vi "Format StateReasonType_LVXML.vi"(8 "error in (no error)":errorcluster, 10 "xmlData in":T2, 11 "AWS_EC2 in":refnum<class "AWS_EC2.lvclass">) -> (0 "error out":errorcluster, 2 "StateReasonType":T3, 3 "AWS_EC2 out":refnum<class "AWS_EC2.lvclass">)   [LabVIEW 2014, in "AWS_EC2.lvlib" / "AWS_EC2.lvclass"]
uses:
  AWS_EC2.lvclass
  EC2 Datatypes/StateReasonType.ctl
  lv-xml-parser/r0/trunk/VI Source/EventType.ctl
  AWS_EC2.lvlib
  lv-xml-parser/r0/trunk/VI Source/LV XML Parser.lvlib
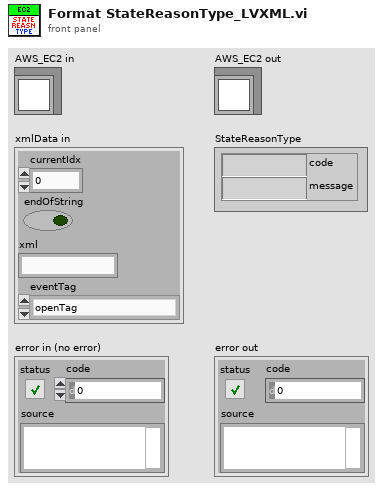
[diagram p1: front panel]
types:
  T1 = typedef "LV XML Parser.lvlib/EventType.ctl" = enum16{"openTag", "endOpenTag", "closeTag", "comment", "endComment", "endOfFile", "attribute", "startXml"}
  T2 = cluster{"currentIdx":i32, "endOfString":bool, "xml":string, "eventTag":T1}
  T3 = typedef "AWS_EC2.lvlib/StateReasonType.ctl" = cluster{"code":string, "message":string}
  T4 = cluster{"namespaceUri":string, "localName":string}
  T5 = cluster{"Attributes":cluster{"localName":string, "namespaceUri":string, "value":string}[], "localName":string, "namespaceUri":string, "valueXmlData":cluster{"currentIdx":i32, "endOfString":bool, "xml":string, "eventTag":T1}}[]
  T6 = cluster{"Attributes":cluster{"localName":string, "namespaceUri":string, "value":string}[], "localName":string, "namespaceUri":string, "valueXmlData":cluster{"currentIdx":i32, "endOfString":bool, "xml":string, "eventTag":T1}}
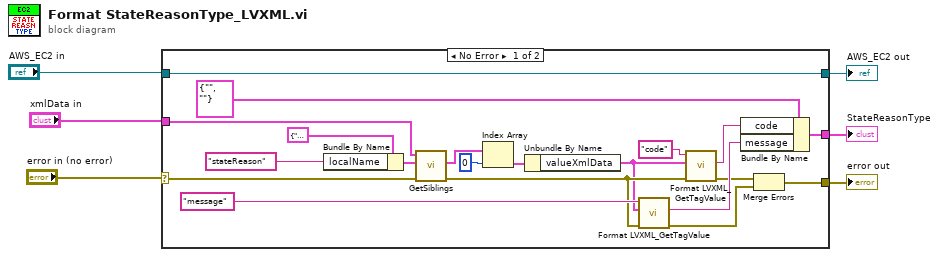
[diagram p0: block diagram]
diagram:
  n1 = case shown="No Error" "error in (no error)" {
    selector: "error in (no error)" -> [w18 w28]
    tunnel: "xmlData in" -> [w19 _]
    tunnel: [w12 w28] -> w2
    tunnel: [w13 _] -> w4
    tunnel: "AWS_EC2 in" -> [w7 w27]
    tunnel: [w7 w27] -> w6
    frame No Error {
      n2 = Bundle By Name(cluster=T4 {"namespaceUri"="", "localName"=""} ("limitToTag"), "localName"="stateReason" ("Tag name")) -> (w25:T4)
      n3 = call "GetSiblings.vi"("error in (no error)"=w18, "limitToTag"=w25, "xmlData"=w19) -> ("error out"=w9:errorcluster, "Siblings"=w22:T5)  [unwired: 7 in]
      n4 = Index Array(array=w22, index=0) -> (element=w21:T6)
      n5 = Unbundle By Name(w21) -> ("valueXmlData"=w8:T2)
      n6 = call "Format LVXML_GetTagValue.vi"("error in (no error)"=w9, "xmlDataIn"=w8, "Tag name"="message") -> ("error out"=w10:errorcluster, "Value"=w15:string)  [unwired: 6 in, 1 out]
      n7 = call "Format LVXML_GetTagValue.vi"("error in (no error)"=w9, "xmlDataIn"=w8, "Tag name"="code") -> ("error out"=w11:errorcluster, "Value"=w14:string)  [unwired: 6 in, 1 out]
      n8 = Bundle By Name(cluster=T3 {"code"="", "message"=""} ("StateReasonType"), "code"=w14, "message"=w15) -> (w13:T3)
      n9 = Merge Errors(w11, w10) -> (w12:errorcluster)
    }
    frame Error {
    }
  }
  "AWS_EC2 out" <- w6
  "StateReasonType" <- w4
  "error out" <- w2
